vi "Sensor Interface - Fire Deposit.vi"(8 "error in (no error)":errorcluster, 10 "Deposit Change":bool, 11 "UE Data Container":T1) -> (0 "error out":errorcluster)   [LabVIEW 2017]
doc: "Generates Deposit change user event."
uses:
  Shared Data/User Events/UE Data Container.ctl
  Error Handler/Controls/Error Data.ctl
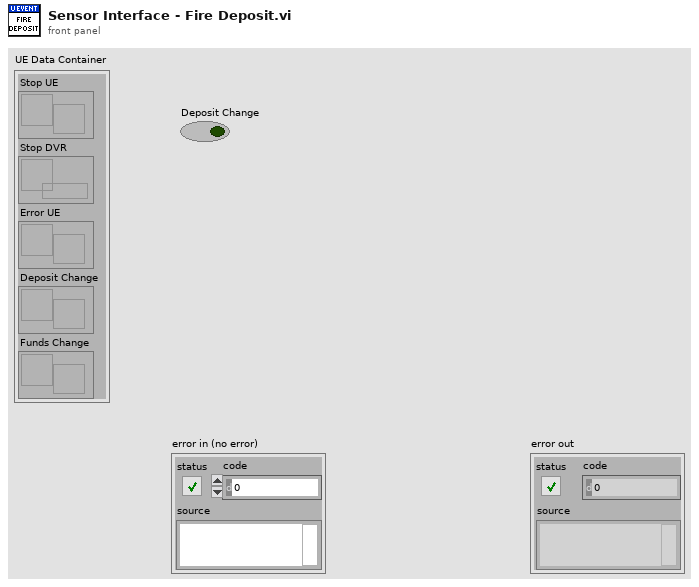
[diagram p1: front panel]
types:
  T1 = typedef "UE Data Container.ctl" = cluster{"Stop UE":refnum<user-event>, "Stop DVR":refnum<data-value>, "Error UE":refnum<user-event>, "Deposit Change":refnum<user-event>, "Funds Change":refnum<user-event>}
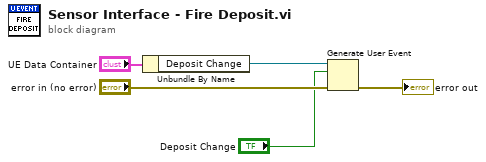
[diagram p0: block diagram]
diagram:
  n1 = Unbundle By Name("UE Data Container") -> ("Deposit Change"=w4:refnum<user-event>)
  n2 = Generate User Event(user event=w4, event data cluster="Deposit Change", error in="error in (no error)") -> (error out=→"error out":errorcluster)  [unwired: 1 in, 1 out]
